vi "State Machine with Intialization.vi"() -> ()   [LabVIEW 2022 SP3]
panel:
  in  "Numeric 2":dbl
  in  "Numeric":dbl
  in  "Fail Check":bool
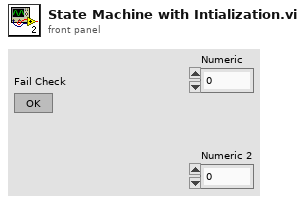
[diagram p1: front panel]
types:
  T1 = enum16{"Intialize", "Temprature Control", "Pressure Control", "Fail Check", "Fail State"}
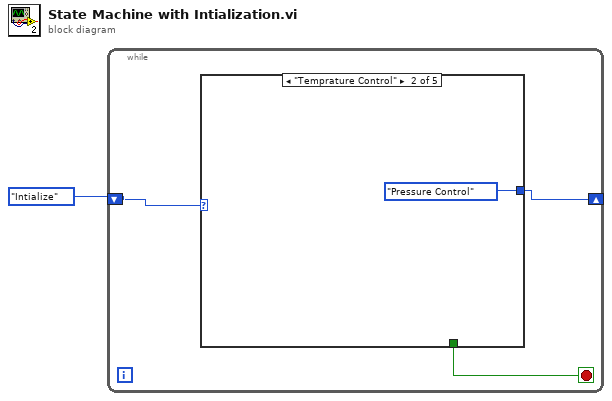
[diagram p0: block diagram]
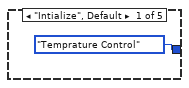
[diagram p2: hidden frame]
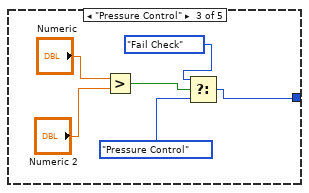
[diagram p3: hidden frame]
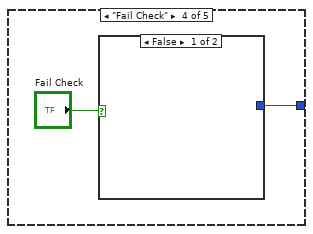
[diagram p4: hidden frame]
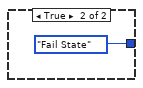
[diagram p5: hidden frame]
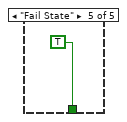
[diagram p6: hidden frame]
diagram:
  n1 = while {
    shift-right: [w3] -> _
    shift-left: T1."Intialize" -> [w4]
    stop <- w2 stop-if-true
    n2 = case shown="\"Temprature Control\"" w4 {
      tunnel: [T1."Temprature Control" T1."Pressure Control" w7 w14 _] -> w3
      tunnel: [_ _ _ _ TRUE] -> w2
      frame "Intialize", Default {
      }
      frame "Temprature Control" {
      }
      frame "Pressure Control" {
        n3 = Greater?(x="Numeric", y="Numeric 2") -> (0:w10:bool)
        n4 = Select(t=T1."Fail Check", s=w10, f=T1."Pressure Control") -> (s? t:f=w7:T1)
      }
      frame "Fail Check" {
        n5 = case shown="False" "Fail Check" {
          tunnel: [_ T1."Fail State"] -> w14
          frame False {
          }
          frame True {
          }
        }
      }
      frame "Fail State" {
      }
    }
  }
